vi "optionsAcq_channel_PD_tempVariable.vi"(8 "error in (no error)":errorcluster, 11 "OSAchannel in":refnum<class "OSAchannel.lvclass">) -> (0 "error out":errorcluster, 3 "OSAchannel out":refnum<class "OSAchannel.lvclass">)   [LabVIEW 2010, in "OSAchannel.lvclass"]
uses:
  OSAchannel.lvclass
  _dll/LVLib/FTSLib.lvlib
panel:
  out "FTSLib_status":i32
  out "auto read":bool
  in  "auto":bool
  in  "readWrite":enum16{"read", "write"}(ring)
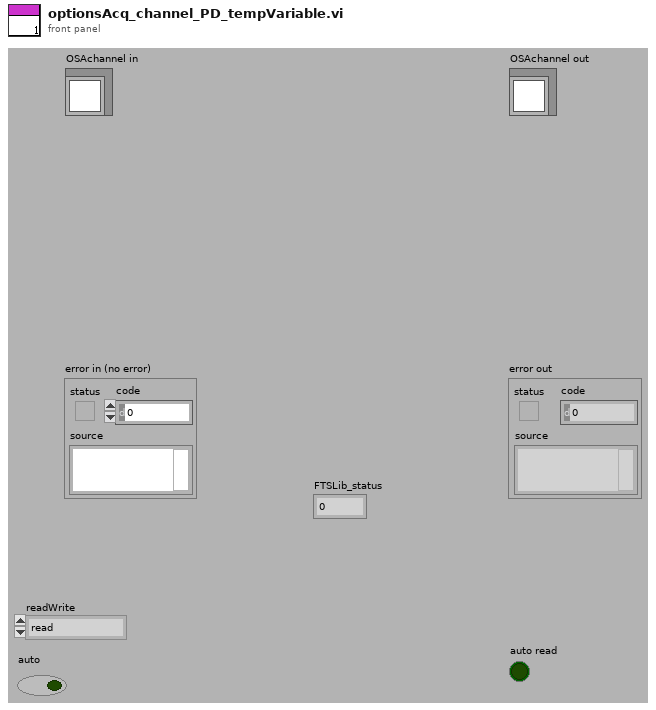
[diagram p1: front panel]
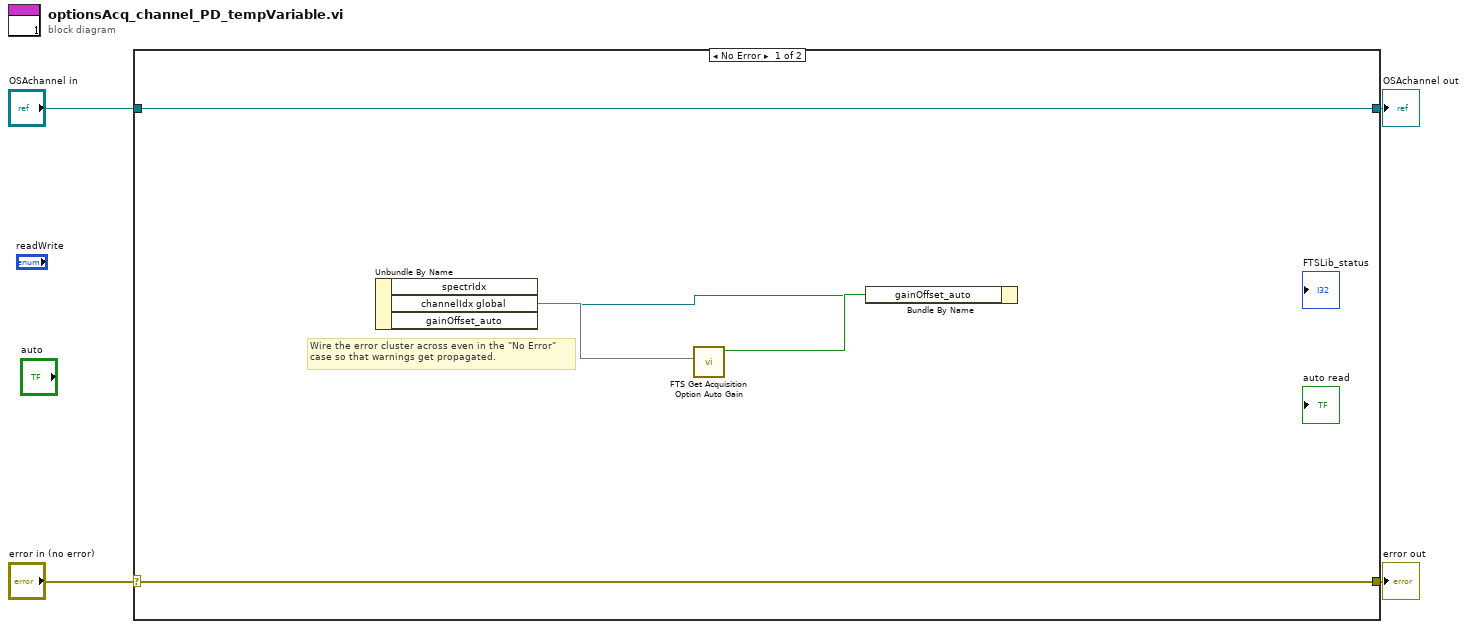
[diagram p0: block diagram]
diagram:
  n1 = case shown="No Error" "error in (no error)" {
    selector: "error in (no error)" -> [w9 w12]
    tunnel: [w9 w12] -> w3
    tunnel: [w10 w11] -> w1
    tunnel: "OSAchannel in" -> [w10 w11]
    frame No Error {
      # "Wire the error cluster across even in the \"No Error\"\ncase so that warnings get propagated."
      n2 = Unbundle By Name() -> (w6:refnum<class "OSAchannel.lvclass">, "channelIdx global"=w8, "gainOffset_auto"=w5)  [unwired: 1 out]
      n3 = call "FTS Get Acquisition Option Auto Gain.vi"("channel"=w8) -> ("function return"=w7:bool)  [unwired: 9 in, 1 out]
      n4 = Bundle By Name(cluster=w6, "gainOffset_auto"=w7) -> ()  [unwired: 1 out]
    }
    frame Error {
    }
  }
  "error out" <- w3
  "OSAchannel out" <- w1
